vi "Overhead_Factor.vi"(1 "Current Overhead Factor In":dbl format="%.1f", 2 "Sum of Ideal times (Sec)":dbl, 3 "Sum of Actual times (Sec)":dbl, 4 "Mode":T1) -> (0 "Current Overhead Factor":dbl format="%.1f")   [LabVIEW 2011]
uses:
  Controls/Overhead.ctl
panel:
  out "Ideal Register":dbl
  out "Actual Register":dbl
  out "Unclamped Factor":dbl format="%.2f"
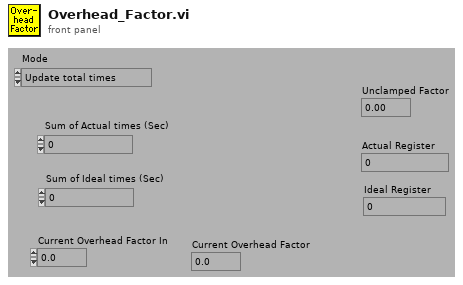
[diagram p1: front panel]
types:
  T1 = typedef "Overhead.ctl" = enum16{"Update total times", "Read Current Overhead", "Re Scale totals to 3 hrs", "Initialise totals to 3hr"}
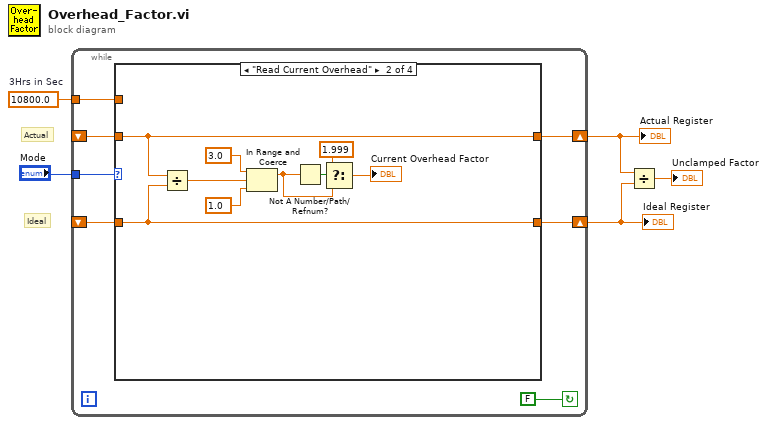
[diagram p0: block diagram]
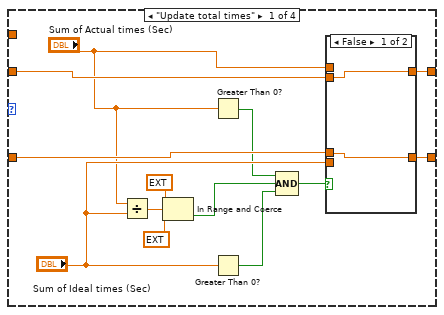
[diagram p2: hidden frame]
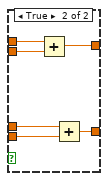
[diagram p3: hidden frame]
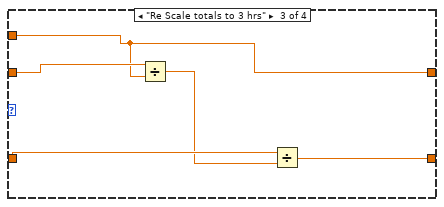
[diagram p4: hidden frame]
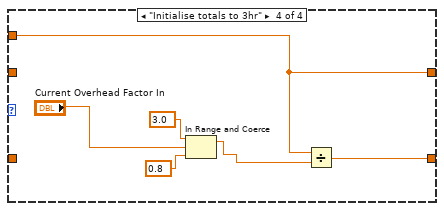
[diagram p5: hidden frame]
diagram:
  w4 = 10800.0  # 3Hrs in Sec
  # "Actual"
  # "Ideal"
  n1 = while {
    tunnel: w4 -> [w7]
    tunnel: "Mode" -> [w12]
    shift-left: _ -> [w9]
    shift-right: [w8] -> w2
    shift-left: _ -> [w11]
    shift-right: [w10] -> w3
    stop <- FALSE continue-if-true
    n2 = case shown="\"Read Current Overhead\"" w12 {
      tunnel: w11 -> [w25 w42 w47 _]
      tunnel: [w24 w42 w43 w49] -> w10
      tunnel: w9 -> [w23 w41 w46 _]
      tunnel: [w22 w41 w44 w50] -> w8
      tunnel: w7 -> [_ _ w43 w49]
      frame "Update total times" {
        n3 = Divide(x="Sum of Actual times (Sec)", y="Sum of Ideal times (Sec)") -> (x/y=w19:dbl)
        n4 = In Range and Coerce(upper limit=ext 4.0 ("hi"), x=w19, lower limit=ext 0.8 ("lo")) -> (In Range?=w14:bool)  [unwired: 1 out]
        n5 = Greater Than 0?(x="Sum of Actual times (Sec)") -> (x > 0?=w15:bool)
        n6 = Greater Than 0?(x="Sum of Ideal times (Sec)") -> (x > 0?=w16:bool)
        n7 = Compound Arithmetic op=AND(w15, w14, w16) -> (w13:bool)
        n8 = case shown="False" w13 {
          tunnel: "Sum of Actual times (Sec)" -> [_ w33]
          tunnel: w25 -> [w27 w32]
          tunnel: [w27 w31] -> w24
          tunnel: w23 -> [w26 w30]
          tunnel: [w26 w29] -> w22
          tunnel: "Sum of Ideal times (Sec)" -> [_ w28]
          frame False {
          }
          frame True {
            n9 = Add(x=w33, y=w32) -> (x+y=w31:dbl)
            n10 = Add(x=w30, y=w28) -> (x+y=w29:dbl)
          }
        }
      }
      frame "Read Current Overhead" {
        n11 = Divide(x=w42, y=w41) -> (x/y=w38:dbl)
        n12 = In Range and Coerce(upper limit=3.0 ("Max"), x=w38, lower limit=1.0 ("Min")) -> (coerced(x)=w35:dbl)  [unwired: 1 out]
        n13 = Not A Number/Path/Refnum?(number/path/refnum=w35) -> (NaN/Path/Refnum?=w37:bool)
        n14 = Select(t=1.999, s=w37, f=w35) -> (s? t:f=→"Current Overhead Factor":dbl)
      }
      frame "Re Scale totals to 3 hrs" {
        n15 = Divide(x=w47, y=w43) -> (x/y=w45:dbl)
        n16 = Divide(x=w46, y=w45) -> (x/y=w44:dbl)
      }
      frame "Initialise totals to 3hr" {
        n17 = In Range and Coerce(upper limit=3.0 ("Max"), x="Current Overhead Factor In", lower limit=0.8 ("Min")) -> (coerced(x)=w48:dbl)  [unwired: 1 out]
        n18 = Divide(x=w49, y=w48) -> (x/y=w50:dbl)
      }
    }
  }
  "Actual Register" <- w3
  "Ideal Register" <- w2
  n19 = Divide(x=w3, y=w2) -> (x/y=→"Unclamped Factor":dbl)
